vi "Register Q.vi"(8 "error in (no error)":errorcluster, 9 "Identities":refnum<class "Identity.lvclass">[](array[class]), 10 "MessageQ":refnum<class "MessageQ.lvclass">, 11 "VolatusAPI in":refnum<class "VolatusAPI.lvclass">) -> (0 "error out":errorcluster, 2 "Q Number":i32, 3 "VolatusAPI out":refnum<class "VolatusAPI.lvclass">)   [LabVIEW 2020, in "Volatus.lvlib" / "VolatusAPI.lvclass"]
uses:
  VolatusAPI.lvclass
  Q Info.ctl
  VolatusAPI.lvclass/VolatusAPI.ctl
  Registered Q.ctl
  Identity/Identity.lvclass
  MessageQ/MessageQ.lvclass
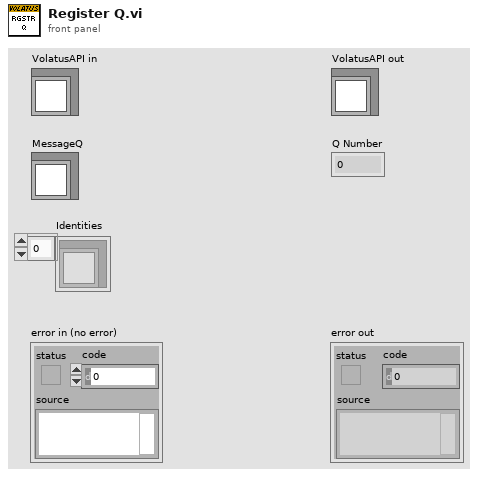
[diagram p1: front panel]
types:
  T1 = typedef "Volatus.lvlib/VolatusAPI.lvclass/Q Info.ctl" = cluster{"Number":i32, "Notifiers":refnum<notifier>[]}
  T2 = typedef "Volatus.lvlib/VolatusAPI.lvclass/Registered Q.ctl" = cluster{"Q":refnum<class "MessageQ.lvclass">, "Keys":string[]}
  T3 = typedef "Volatus.lvlib/VolatusAPI.lvclass/MsgQs Ref.ctl" = cluster{"Keys":map{string, T1}, "MsgQs":map{i32, T2}, "Next Number":i32}
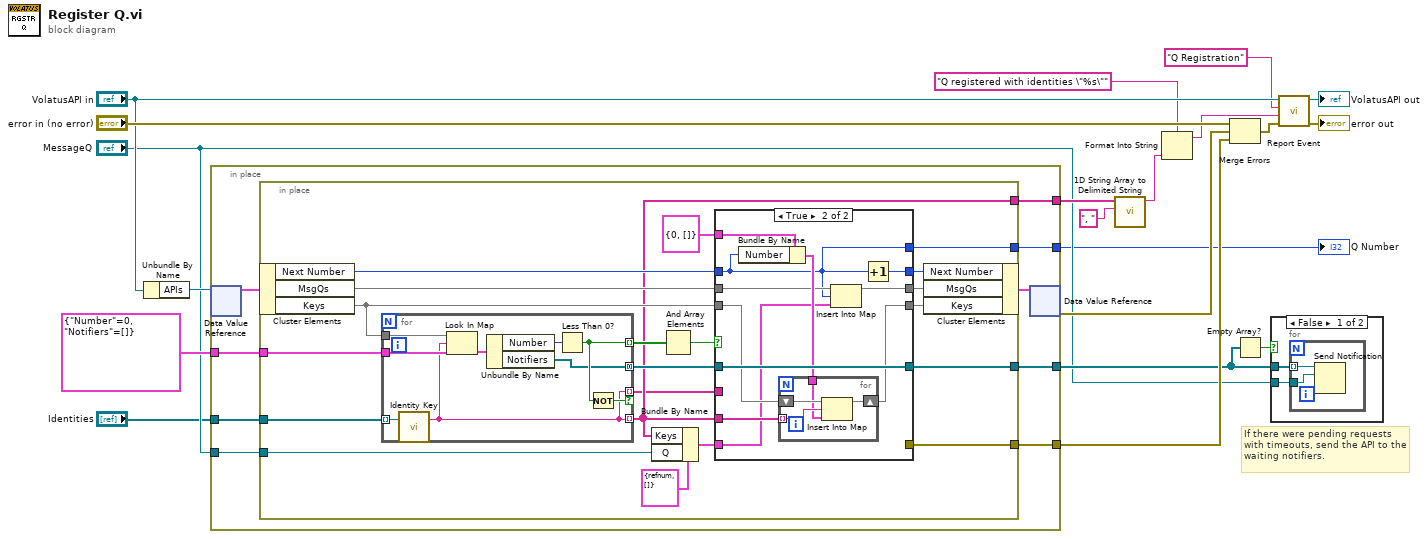
[diagram p0: block diagram]
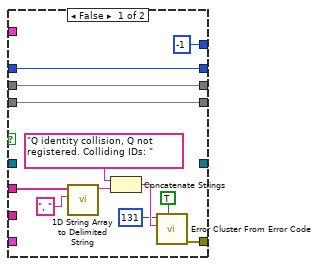
[diagram p3: hidden frame]
diagram:
  # "If there were pending requests with timeouts, send the API to the waiting notifiers."
  n1 = Unbundle By Name("VolatusAPI in") -> ("APIs"=w12:refnum<data-value>)
  n2 = in-place {
    in-place-border: "MessageQ" -> [w28]
    in-place-border: [w27] -> w10
    in-place-border: T1 {"Number"=0, "Notifiers"=[]} ("default value") -> [w26]
    in-place-border: [w24] -> w4
    in-place-border: [w23] -> w7
    in-place-border: [w22] -> w2
    in-place-border: "Identities" -> [w21]
    n3 = in-place-dvr #1(w12) -> (w29:T3)  [unwired: 1 out]
    n4 = in-place {
      in-place-border: w28 -> [w36]
      in-place-border: [w38] -> w27
      in-place-border: w26 -> [w48]
      in-place-border: [w41] -> w24
      in-place-border: [w32] -> w23
      in-place-border: [w31] -> w22
      in-place-border: w21 -> [w30]
      n5 = in-place-cluster #2(w29) -> ("Next Number"=w43:i32, "MsgQs"=w44:map{i32, T2}, "Keys"=w45:map{string, T1})
      n6 = for {
        tunnel: w30 -> [w58] mode=indexing
        tunnel: w45 -> [w57]
        tunnel: [w53] -> w49 mode=indexing
        tunnel: [w50] -> w38 mode=indexing
        tunnel: [w50] -> w33 mode=indexing if=w52
        tunnel: w48 -> [w56]
        tunnel: [w51] -> w46 mode=concatenating
        n7 = call "Identity Key.vi"("Identity in"=w58) -> ("Identity Key"=w50:string)  [unwired: 2 in]
        n8 = Look In Map(map=w57, key=w50, default value=w56) -> (value=w55:T1)  [unwired: 1 out]
        n9 = Unbundle By Name(w55) -> ("Number"=w54:i32, "Notifiers"=w51:refnum<notifier>[])
        n10 = Less Than 0?(x=w54) -> (x < 0?=w53:bool)
        n11 = Not(x=w53) -> (.not. x?=w52:bool)
      }
      n12 = Bundle By Name(cluster=T2 {"Q"=refnum, "Keys"=[]} ("Registered API"), "Keys"=w38, "Q"=w36) -> (w35:T2)
      n13 = And Array Elements(Boolean array=w49) -> (logical AND=w47:bool)
      n14 = case shown="True" w47 {
        tunnel: w46 -> [_ w80]
        tunnel: w45 -> [w68 w78]
        tunnel: w44 -> [w69 w74]
        tunnel: w43 -> [w70 w71]
        tunnel: [w70 w81] -> w42
        tunnel: [_ w80] -> w41
        tunnel: T1 {"Number"=0, "Notifiers"=[]} ("API Info") -> [_ w79]
        tunnel: [w68 w77] -> w39
        tunnel: w38 -> [_ w75]
        tunnel: w35 -> [_ w72]
        tunnel: [w69 w73] -> w34
        tunnel: w33 -> [w61 _]
        tunnel: [w60 _] -> w32
        tunnel: [-1 ("Next Number") w71] -> w31
        frame False {
          n15 = call <vilib>:"1D String Array to Delimited String.vi"("delimiter"=", ", "string array"=w61) -> ("delimited string"=w66:string)  [unwired: 9 in]
          n16 = Concatenate Strings("Q identity collision, Q not registered. Colliding IDs: ", w66) -> (w67:string)
          n17 = call <vilib>:"Error Cluster From Error Code.vi"("show call chain? (False)"=TRUE, "error message (\"\")"=w67, "error code (0)"=131) -> ("error out"=w60:errorcluster)  [unwired: 6 in]
        }
        frame True {
          n18 = Bundle By Name(cluster=w79, "Number"=w71) -> (w76:T1)
          n19 = for {
            tunnel: w75 -> [w85] mode=indexing
            shift-right: [w83] -> w77
            shift-left: w78 -> [w84]
            tunnel: w76 -> [w82]
            n20 = Insert Into Map(map in=w84, key=w85, value=w82) -> (map out=w83:map{string, T1})  [unwired: 2 out]
          }
          n21 = Insert Into Map(map in=w74, key=w71, value=w72) -> (map out=w73:map{i32, T2})  [unwired: 2 out]
          n22 = Increment(x=w71) -> (x+1=w81:i32)
        }
      }
      n23 = in-place-cluster #2("Next Number"=w42, "MsgQs"=w34, "Keys"=w39) -> (w25:T3)
    }
    n24 = in-place-dvr #1(w25) -> (w6:errorcluster)  [unwired: 1 out]
  }
  "Q Number" <- w2
  n25 = call <vilib>:"1D String Array to Delimited String.vi"("delimiter"=", ", "string array"=w10) -> ("delimited string"=w16:string)  [unwired: 9 in]
  n26 = Format Into String(format string="Q registered with identities \"%s\"", w16) -> (resulting string=w15:string)  [unwired: 2 in, 1 out]
  n27 = Merge Errors("error in (no error)", w6, w7) -> (w14:errorcluster)
  n28 = Empty Array?(array=w4) -> (empty?=w5:bool)
  n29 = case shown="False" w5 {
    tunnel: w4 -> [w87 _]
    tunnel: "MessageQ" -> [w86 _]
    frame False {
      n30 = for {
        tunnel: w87 -> [w89] mode=indexing
        tunnel: w86 -> [w88]
        n31 = Send Notification(notification=w88, notifier=w89) -> ()  [unwired: 1 in, 2 out]
      }
    }
    frame True {
    }
  }
  n32 = call "Report Event.vi"("error in (no error)"=w14, "Message"=w15, "Context"="Q Registration", "VolatusAPI in"="VolatusAPI in") -> ("error out"=→"error out":errorcluster, "VolatusAPI out"=→"VolatusAPI out":refnum<class "VolatusAPI.lvclass">)  [unwired: 6 in]
